vi "JSONPath to EXCEL.vi"(8 "error in":errorcluster, 11 "JSONPath":string) -> (0 "error out":errorcluster, 3 "Childs":string[](array[string]))   [LabVIEW 2024, in "Config from EXCEL.lvclass"]
uses:
  Config from EXCEL.lvclass
  Config from EXCEL.lvclass/Config from EXCEL.ctl
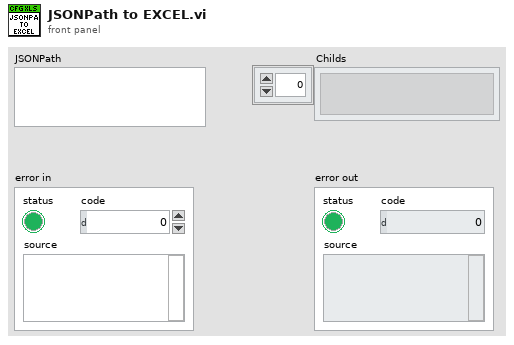
[diagram p1: front panel]
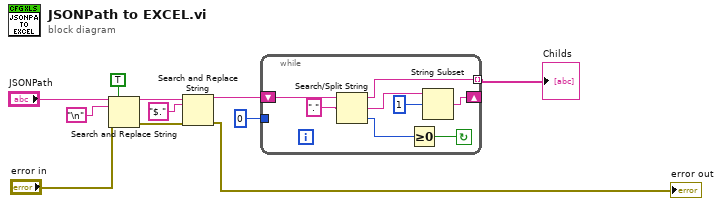
[diagram p0: block diagram]
diagram:
  n1 = Search and Replace String(replace all?=TRUE ("replace all? (F)"), input string="JSONPath", search string="\n", error in="error in") -> (result string=w6:string, error out=w4:errorcluster)  [unwired: 4 in, 2 out]
  n2 = Search and Replace String(input string=w6, search string="$." ("search string/char (-)"), error in=w4) -> (result string=w3:string, error out=→"error out":errorcluster)  [unwired: 5 in, 2 out]
  n3 = while {
    tunnel: [w16] -> w1 mode=indexing
    shift-right: [w12] -> _
    shift-left: w3 -> [w19]
    tunnel: 0 ("offset of match") -> [_]
    stop <- w17 continue-if-true
    n4 = Search/Split String(string=w19, search string/char (-)=".") -> (substring before match=w16:string, match + rest of string=w15:string, offset of match=w14:i32)  [unwired: 1 in]
    n5 = Greater Or Equal To 0?(x=w14) -> (x >= 0?=w17:bool)
    n6 = String Subset(string=w15, offset (0)=1) -> (substring=w12:string)  [unwired: 1 in]
  }
  "Childs" <- w1
